vi "Zapis danych do pliku txt.vi"(0 "Dane zapisane z przejazdu \n(współrzędne, prędkości, azymut)":path=path "C:/Users/User/Desktop/dane autozapis.txt", 3 "Długość geograficzna - GPS":dbl, 4 "Szerokośc geograficzna - GPS":dbl, 5 "Azymut [stopnie]":dbl) -> ()   [LabVIEW 2015, in "Biblioteka moduł map v3.lvlib" / "Pomocnicze.lvlib"]
doc: "Plik zapisuje dane w kolumnach w nastepującej kolejności:\nVr koła[obr/min], Vl koła[obr/min], Długość geograficzna, Szerokość geograficzna, Azymut[stopnie]"
uses:
  Pomocnicze.lvlib
  <vilib>/Utility/file.llb/Read Delimited Spreadsheet (DBL).vi
  <vilib>/Utility/file.llb/Write Delimited Spreadsheet (DBL).vi
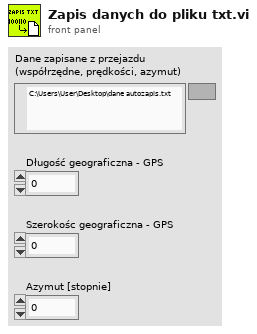
[diagram p1: front panel]
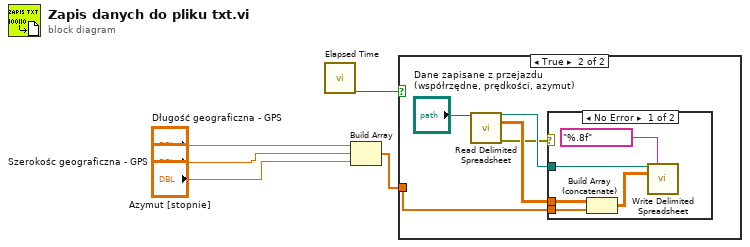
[diagram p0: block diagram]
diagram:
  n1 = call "Elapsed Time"() -> ("Time has Elapsed"=w4:bool)  [unwired: 12 in, 7 out]
  n2 = Build Array("Długość geograficzna - GPS", "Szerokośc geograficzna - GPS", "Azymut [stopnie]") -> (w5:dbl[])
  n3 = case shown="True" w4 {
    tunnel: w5 -> [_ w7]
    frame False {
    }
    frame True {
      n4 = call-poly <vilib>:"Read Delimited Spreadsheet.vi"("file path (dialog if empty)"="Dane zapisane z przejazdu \n(współrzędne, prędkości, azymut)") -> ("new file path (Not A Path if cancelled)"=w9:path, "all rows"=w8:dbl[][], "error out"=w6:errorcluster)  [unwired: 9 in, 3 out]
      n5 = case shown="No Error" w6 {
        tunnel: w9 -> [w14 _]
        tunnel: w8 -> [w13 _]
        tunnel: w7 -> [w12 _]
        frame No Error {
          n6 = Build Array (concatenate)(w13, w12) -> (w11:dbl[][])
          n7 = call-poly <vilib>:"Write Delimited Spreadsheet.vi"("file path (dialog if empty)"=w14, "format (%.3f)"="%.8f", "2D data"=w11) -> ()  [unwired: 11 in, 2 out]
        }
        frame Error {
        }
      }
    }
  }
